vi "Apply Configuration.vi"(8 "error in (no error)":errorcluster, 11 "PXIe-5172 Simulated in":refnum<class "PXIe-5172 Simulated.lvclass">) -> (0 "error out":errorcluster, 3 "PXIe-5172 Simulated out":refnum<class "PXIe-5172 Simulated.lvclass">)   [LabVIEW 2023, in "PXIe-5172 Simulated.lvlib" / "PXIe-5172 Simulated.lvclass"]
uses:
  PXIe-5172 Simulated.lvclass
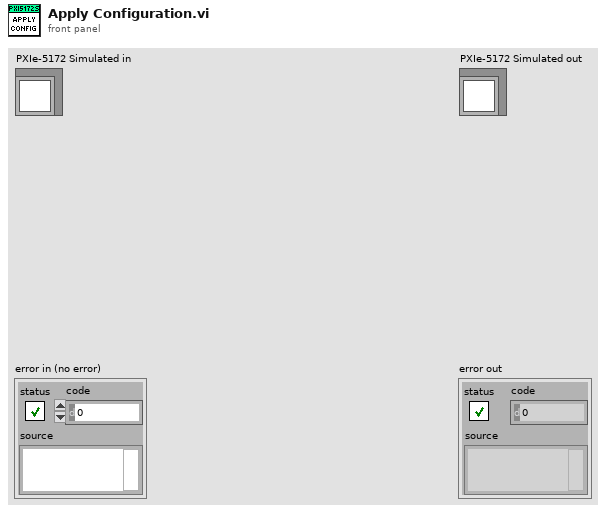
[diagram p1: front panel]
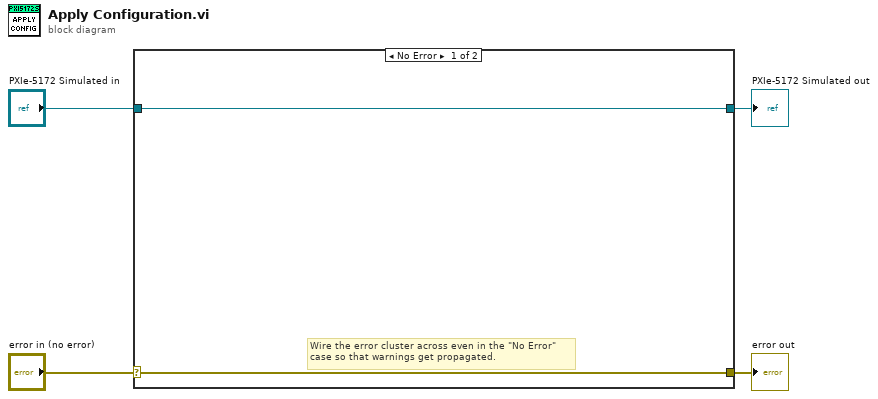
[diagram p0: block diagram]
diagram:
  n1 = case shown="No Error" "error in (no error)" {
    selector: "error in (no error)" -> [w5 w8]
    tunnel: [w5 w8] -> w3
    tunnel: [w6 w7] -> w1
    tunnel: "PXIe-5172 Simulated in" -> [w6 w7]
    frame No Error {
      # "Wire the error cluster across even in the \"No Error\"\ncase so that warnings get propagated."
    }
    frame Error {
    }
  }
  "error out" <- w3
  "PXIe-5172 Simulated out" <- w1
